vi "write_sequential_command.vi"(10 "Number of Sequences":dbl, 11 "Number of Sequential Cycles":dbl) -> (3 "Command Out":string)   [LabVIEW 2015]
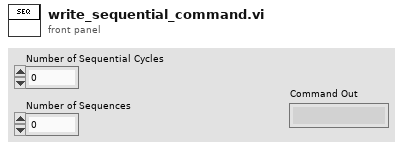
[diagram p1: front panel]
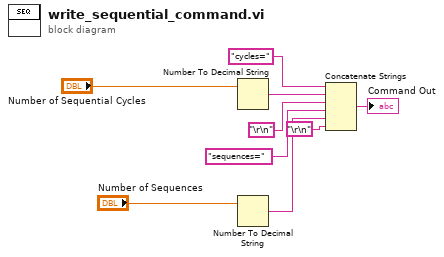
[diagram p0: block diagram]
diagram:
  n1 = Number To Decimal String(number="Number of Sequential Cycles") -> (decimal integer string=w6:string)  [unwired: 1 in]
  n2 = Number To Decimal String(number="Number of Sequences") -> (decimal integer string=w2:string)  [unwired: 1 in]
  n3 = Concatenate Strings("cycles=", w6, "\r\n", "sequences=", w2, "\r\n") -> (→"Command Out":string)
